vi "voltage phase conv SM.vi"() -> ()   [LabVIEW 2019]
uses:
  <vilib>/Utility/file.llb/Write Delimited Spreadsheet (DBL).vi
panel:
  in  "Stop Button":bool
  out "Current pixel":dbl=591.0
  in  "Max pixel":i32=590
  in  "Mask B Calibration Path":path=path "G:/My Drive/ansom/Data/THz 1/pulse shaping/SLM voltage calibration 20 July 2021/Mask B voltage transmission.txt"
  in  "Mask A Calibration Path":path=path "G:/My Drive/ansom/Data/THz 1/pulse shaping/SLM voltage calibration 20 July 2021/Mask A voltage transmission.txt"
  in  "Mask B Data folder":path=path "G:/My Drive/ansom/Data/THz 1/pulse shaping/SLM voltage calibration 20 July 2021/Mask_B_phase_voltage"
  in  "Mask A Data folder":path=path "G:/My Drive/ansom/Data/THz 1/pulse shaping/SLM voltage calibration 20 July 2021/Mask_A_phase_voltage"
  in  "Starting pixel":dbl=518.0 format="%#_13g"
  in  "START":bool
  # "Inputs"
  # "Insert file paths to SLM calibration output .txt files"
  # "Insert folder paths to tell the program where to save voltage/phase .txt files"
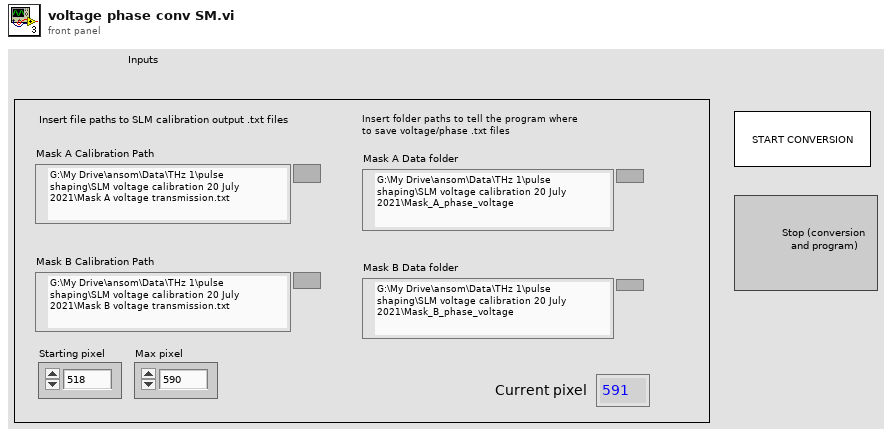
[diagram p1: front panel]
types:
  T1 = enum32{"Invalid", "Standard", "Closed", "Hidden", "Minimized", "Maximized"}
  T2 = enum32{"invalid app kind", "Development System", "Run Time System", "Student Edition", "Embedded LabVIEW", "Evaluation", "Custom"}
  T3 = cluster{"Core":cluster{"Current VI Reference":refnum<vi>, "Close Panel on Exit?":bool}, "Your Boolean data":bool, "Your string data":string}
  T4 = cluster{"Current VI Reference":refnum<vi>, "Close Panel on Exit?":bool}
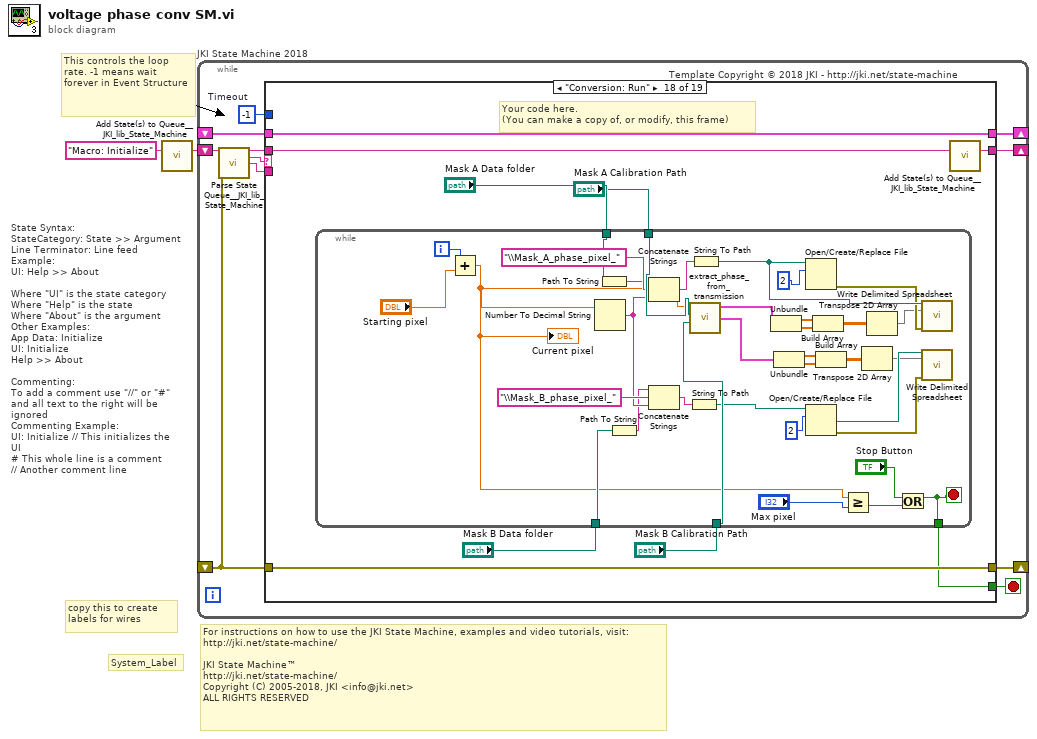
[diagram p0: block diagram]
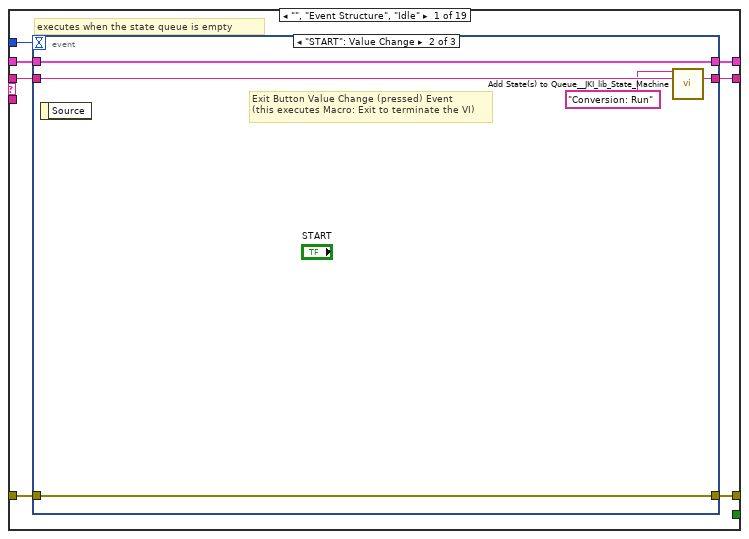
[diagram p2: hidden frame]
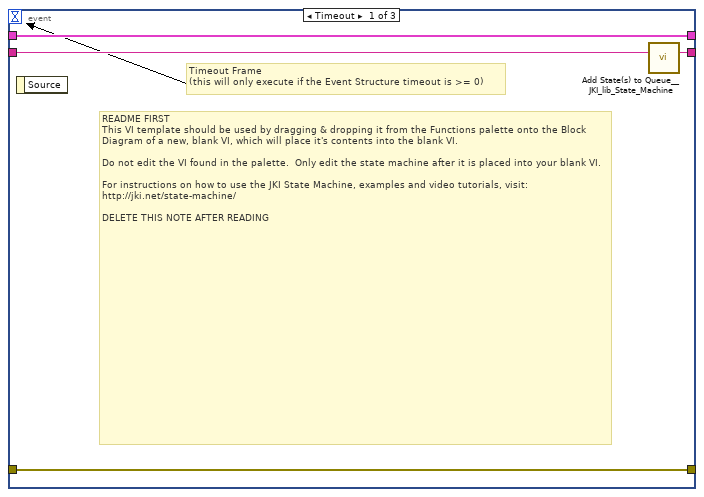
[diagram p3: hidden frame]
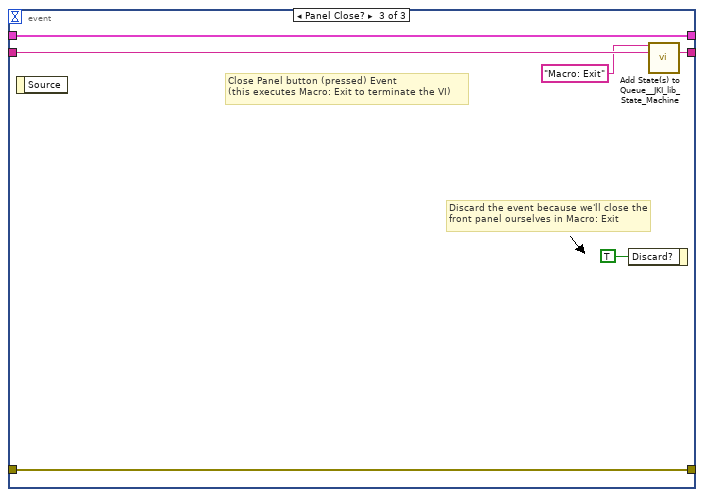
[diagram p4: hidden frame]
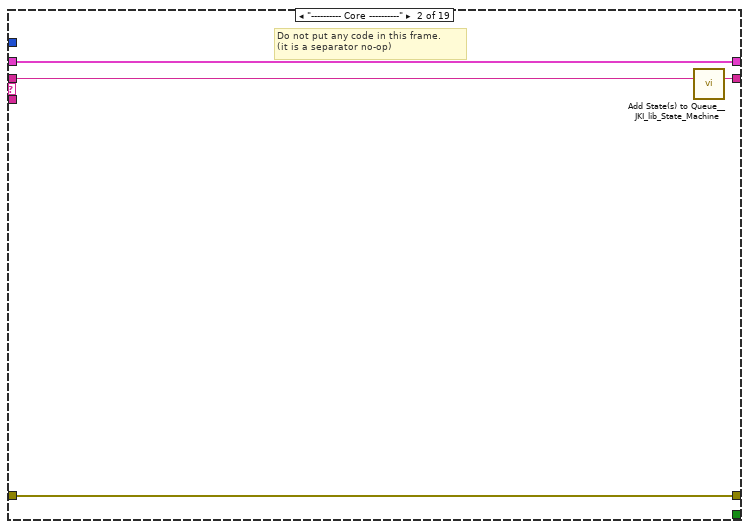
[diagram p5: hidden frame]
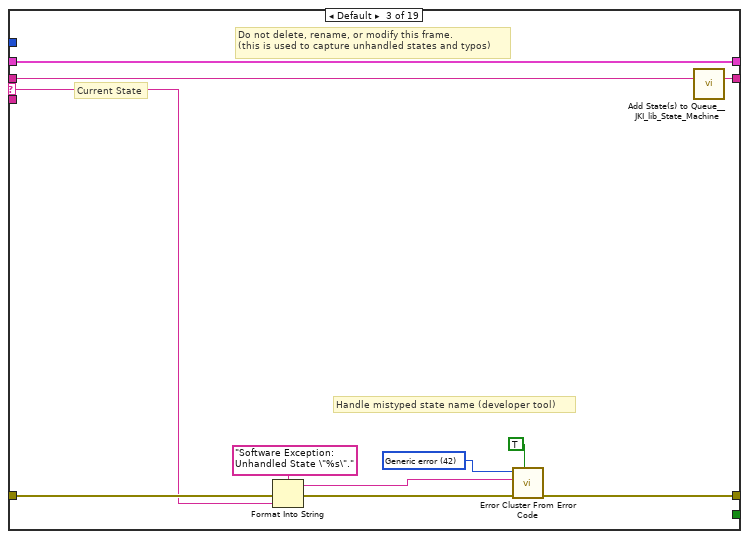
[diagram p6: hidden frame]
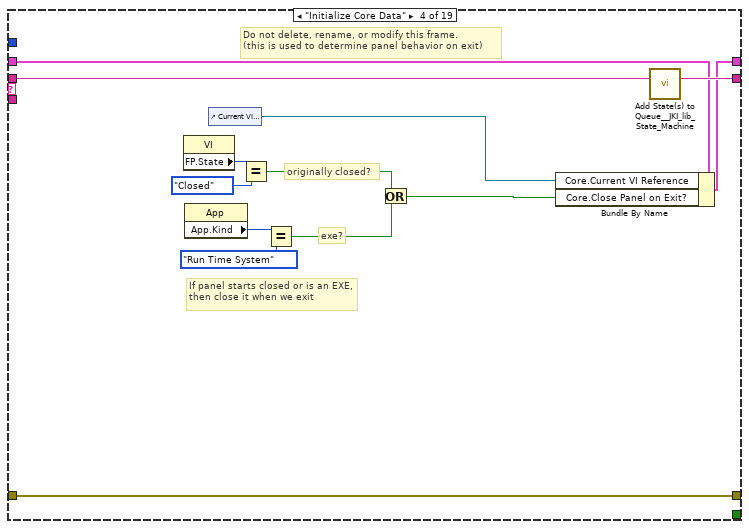
[diagram p7: hidden frame]
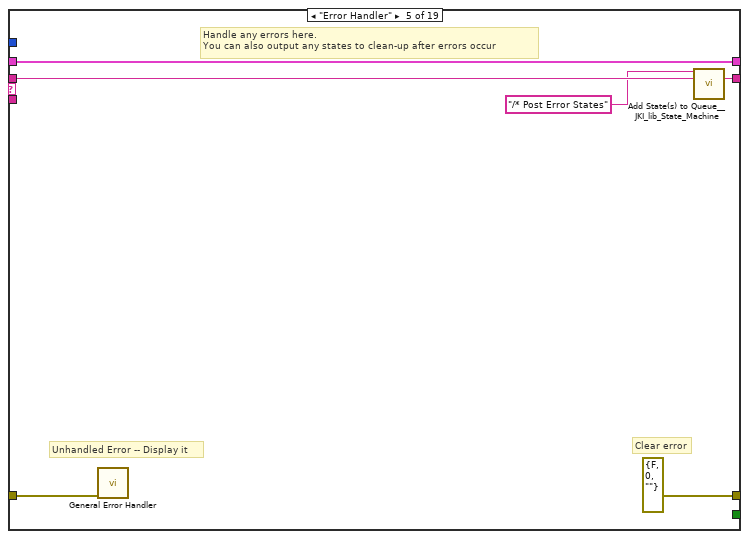
[diagram p8: hidden frame]
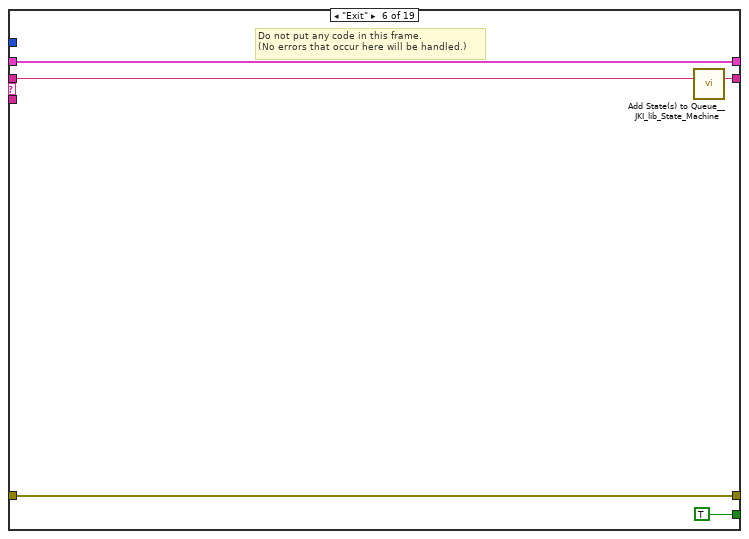
[diagram p9: hidden frame]
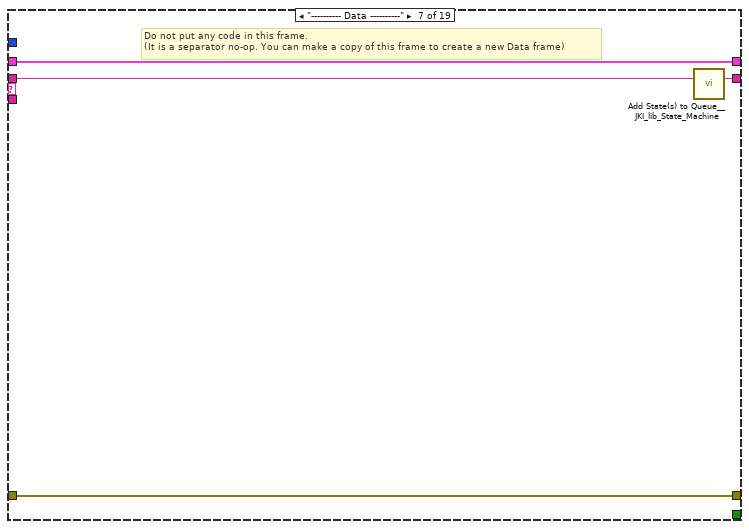
[diagram p10: hidden frame]
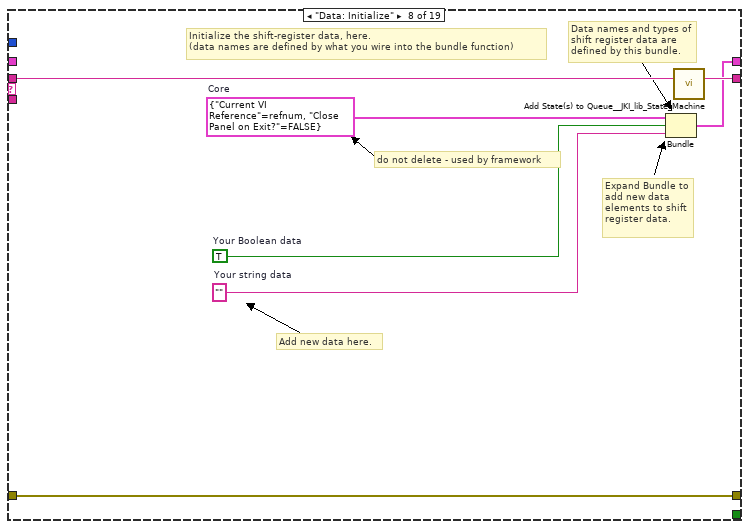
[diagram p11: hidden frame]
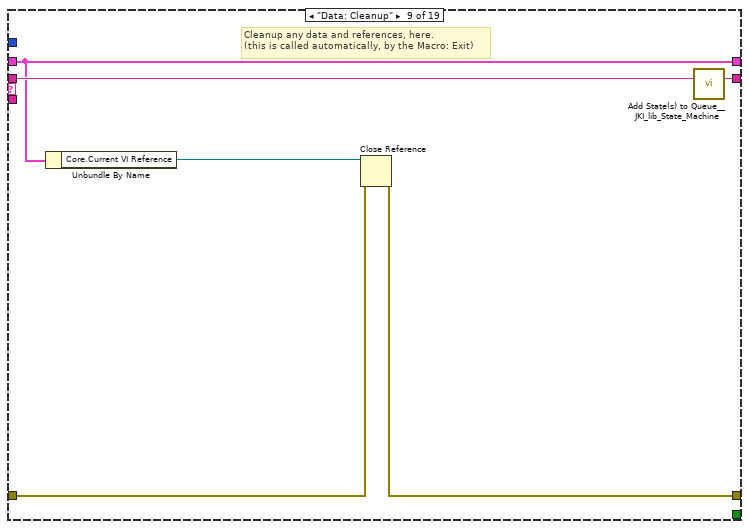
[diagram p12: hidden frame]
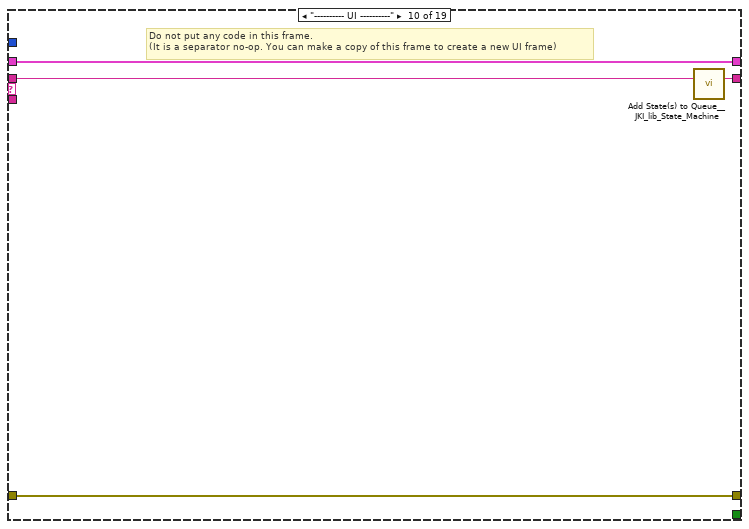
[diagram p13: hidden frame]
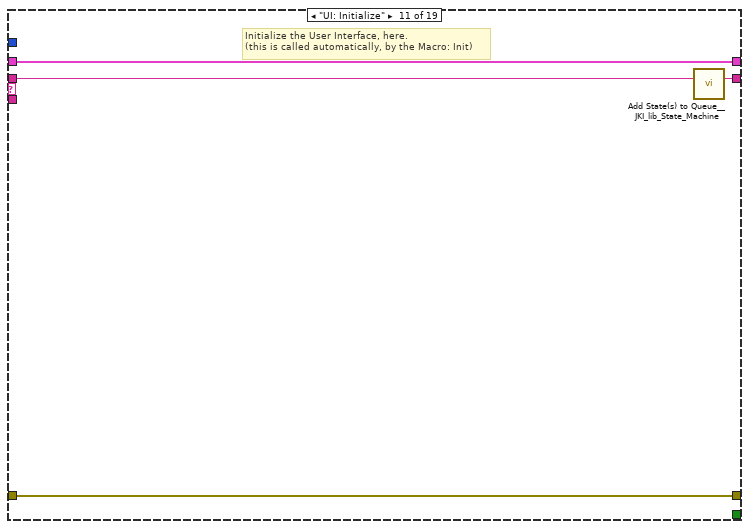
[diagram p14: hidden frame]
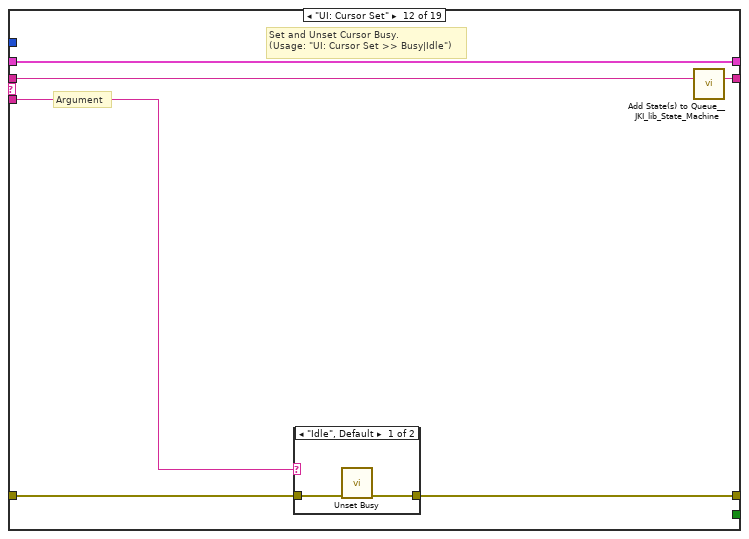
[diagram p15: hidden frame]
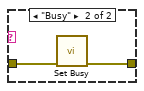
[diagram p16: hidden frame]
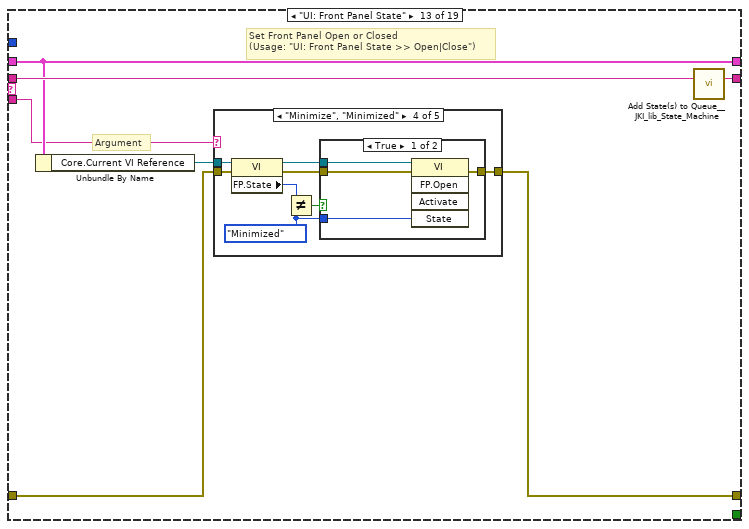
[diagram p17: hidden frame]
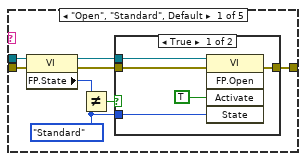
[diagram p18: hidden frame]
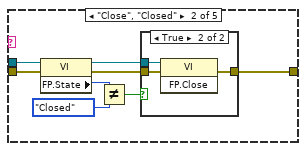
[diagram p20: hidden frame]
diagram:
  # "For instructions on how to use the JKI State Machine, examples and video tutorials, visit:\nhttp://jki.net/state-machine/\n\nJKI State Machine™\nhttp://jki.net/state-machine/\nCopyright (C) 2005-2018, JKI <info@jki.net>\nALL RIGHTS RESERVED"
  # "State Syntax:\nStateCategory: State >> Argument\nLine Terminator: Line feed\nExample:\nUI: Help >> About\n\nWhere \"UI\" is the state category\nWhere \"Help\" is the state\nWhere \"About\" is the argument\nOther Examples:\nApp Data: Initialize\nUI: Initialize\nHelp >> About\n\nCommenting:\nTo add a comment use \"//\" or \"#\" and all text to the right will be ignored\nCommenting Example:\nUI: Initialize // This initializes the UI\n# This whole line is a comment\n// Another comment line"
  # "copy this to create labels for wires"
  # "This controls the loop rate. -1 means wait forever in Event Structure"
  # "System_Label"
  n1 = call <vilib>:"Add State(s) to Queue__JKI_lib_State_Machine.vi"("State(s) in (\"\")"="Macro: Initialize") -> ("States Out"=w2:string)  [unwired: 14 in]
  n2 = while "JKI State Machine 2018" {
    shift-right: [w6] -> _
    shift-left: _ -> [w5]
    shift-right: [w9] -> _
    shift-left: _ -> [w3]
    shift-right: [w8] -> _
    shift-left: w2 -> [w10]
    stop <- w7 stop-if-true
    w4 = -1  # Timeout
    # "Template Copyright © 2018 JKI - http://jki.net/state-machine"
    n3 = call <vilib>:"Parse State Queue__JKI_lib_State_Machine.vi"("State Queue"=w10, "Error In (no error)"=w3) -> ("Remaining States"=w12:string, "Current State"=w13:string, "Arguments"=w11:string)  [unwired: 11 in]
    n4 = case shown="\"Conversion: Run\"" w13 {
      selector: w13 -> [_ _ w40 _ _ _ _ _ _ _ _ _ _ _ _ _ _ _ _]
      tunnel: w12 -> [w20 w39 w44 w63 w69 w74 w78 w85 w91 w95 w99 w105 w116 w185 w190 w200 w204 w213 w251]
      tunnel: w11 -> [_ _ _ _ _ _ _ _ _ _ _ w100 w110 _ _ _ _ _ _]
      tunnel: w5 -> [w18 w36 w42 w56 w66 w72 w75 _ w86 w92 w97 w103 w112 w182 w187 w197 w201 w210 w248]
      tunnel: [w17 w37 w46 w60 errorcluster {"status"=FALSE, "code"=0, "source"=""} ("error out") w71 w76 w82 w87 w93 w96 w101 w113 w183 w188 w198 w202 w211 w249] -> w9
      tunnel: w3 -> [w16 w37 w45 w60 w65 w71 w76 w82 w88 w93 w96 w102 w114 w183 w188 w198 w202 w211 w249]
      tunnel: [w19 w38 w43 w62 w68 w73 w77 w84 w90 w94 w98 w104 w115 w184 w189 w199 w203 w212 w250] -> w8
      tunnel: [_ _ _ _ _ TRUE _ _ _ _ _ _ _ _ _ _ _ w205 _] -> w7
      tunnel: [w15 w36 w42 w61 w66 w72 w75 w83 w86 w92 w97 w103 w112 w182 w187 w197 w201 w210 w248] -> w6
      tunnel: w4 -> [w14 _ _ _ _ _ _ _ _ _ _ _ _ _ _ _ _ _ _]
      frame "", "Event Structure", "Idle" {
        # "executes when the state queue is empty"
        n5 = event shown="[1] \"START\": Value Change" {
          selector: _ -> [_ _ _]
          dyn-events: _ -> [_ _ _]
          timeout: w14 -> [_ _ _]
          tunnel: w20 -> [w24 w29 w35]
          tunnel: [w23 w28 w34] -> w19
          tunnel: w18 -> [w21 w26 w32]
          tunnel: [w22 w27 w33] -> w17
          tunnel: w16 -> [w22 w27 w33]
          tunnel: [w21 w26 w32] -> w15
          event Timeout {
            # "README FIRST\nThis VI template should be used by dragging & dropping it from the Functions palette onto the Block Diagram of a new, blank VI, which will place it's contents into the blank VI.\n\nDo not edit the VI found in the palette.  Only edit the state machine after it is placed into your blank VI.\n\nFor instructions on how to use the JKI State Machine, examples and video tutorials, visit:\nhttp://jki.net/state-machine/\n\nDELETE THIS NOTE AFTER READING"
            # "Timeout Frame\n(this will only execute if the Event Structure timeout is >= 0)"
            n6 = event-data() -> ()  [unwired: 1 in, 1 out]
            n7 = call <vilib>:"Add State(s) to Queue__JKI_lib_State_Machine.vi"("State(s) in (\"\")"=w24) -> ("States Out"=w23:string)  [unwired: 14 in]
          }
          event "START": Value Change {
            # "Exit Button Value Change (pressed) Event\n(this executes Macro: Exit to terminate the VI)"
            n8 = event-data() -> ()  [unwired: 1 in, 1 out]
            n9 = call <vilib>:"Add State(s) to Queue__JKI_lib_State_Machine.vi"("State(s) in Front (\"\")"="Conversion: Run", "State(s) in (\"\")"=w29) -> ("States Out"=w28:string)  [unwired: 13 in]
          }
          event Panel Close? {
            # "Discard the event because we'll close the front panel ourselves in Macro: Exit"
            # "Close Panel button (pressed) Event\n(this executes Macro: Exit to terminate the VI)"
            n10 = event-data() -> ()  [unwired: 1 in, 1 out]
            n11 = event-data("Discard?"=TRUE) -> ()  [unwired: 1 in, 1 out]
            n12 = call <vilib>:"Add State(s) to Queue__JKI_lib_State_Machine.vi"("State(s) in Front (\"\")"="Macro: Exit", "State(s) in (\"\")"=w35) -> ("States Out"=w34:string)  [unwired: 13 in]
          }
        }
      }
      frame "---------- Core ----------" {
        # "Do not put any code in this frame.\n(it is a separator no-op)"
        n13 = call <vilib>:"Add State(s) to Queue__JKI_lib_State_Machine.vi"("State(s) in (\"\")"=w39) -> ("States Out"=w38:string)  [unwired: 14 in]
      }
      frame Default {
        w49 = 42 items=["No error", "Argument error", "Memory is full", "Out of zone", "End of file", "File already open", "Generic file I/O error", "File not found", "File permission error", "Disk is full", "Duplicate path", "Too many files open", "System feature not enabled", "Resource file not found", "Cannot add resource", "Resource not found", "Image not found", "Image memory error", "Pen does not exist", "Config type invalid", "Config token not found", "Config parse error", "Config memory error", "Bad external code format", "Bad external code offset", "External code not present", "Null window", "Destroy window error", "Null menu", "Print aborted", "Bad print record", "Print driver error", "Windows error during printing", "Memory error during printing", "Print dialog error", "Generic print error", "Invalid device refnum", "Device not found", "Device parameter error", "Device unit error", "Cannot open device", "Device call aborted", "Generic error", "Cancelled by user", "Object ID too low", "Object ID too high", "Object not in heap", "Unknown heap", "Unknown object (invalid DefProc)", "Unknown object (DefProc not in table)", "Message out of range", "Invalid (null) method", "Unknown message", "Manager call not supported", "Bad address", "Network operation in progress", "Network operation timed out", "Connection is busy", "Network attribute not supported", "Network error", "Address in use", "System out of memory", "Connection aborted", "Connection refused", "Not connected", "Already connected", "Connection closed", "Initialization error (interapplication manager)", "Bad occurrence", "Wait on unbound occurrence handler", "Occurrence queue overflow", "Datalog type conflict", "Unused", "Unrecognized type (interapplication manager)", "Memory corrupt", "Failed to make temporary DLL", "Old CIN version", "Drag socket not found", "Failed to load drop-object", "Failed to register OLE object", "Failed to release OLE object", "Format specifier type mismatch", "Unknown format specifier", "Too few format specifiers", "Too many format specifiers", "Scan failed", "Newer CIN version", "Error converting to variant", "Runtime menu error", "Password tampered", "Variant attribute not found", "Incompatible variant data type", "Event data is not available", "Event Store is not present", "Occurrence is not found", "Event Queue is not created", "Event info is not available", "Refnum passed is NULL", "Error retrieving Class GUID", "Error retrieving CoClass GUID", "Error retrieving TypeLib GUID.", "Bad built application magic bytes.", "Specific driver is different from the specific driver associated with the Logical Name.", "There is no session opened to the class driver.", "Max Error", "MAX - Error with config objects", "MAX - Error loading configuration", "MAX - Group not supported"]
        # "Current State"
        # "Do not delete, rename, or modify this frame.\n(this is used to capture unhandled states and typos)"
        # "Handle mistyped state name (developer tool)"
        n14 = Format Into String(format string="Software Exception: Unhandled State \"%s\"." ("message"), error in=w45, w40) -> (resulting string=w48:string, error out=w47:errorcluster)  [unwired: 1 in]
        n15 = call <vilib>:"Error Cluster From Error Code.vi"("show call chain? (False)"=TRUE, "error in (no error)"=w47, "error message (\"\")"=w48, "error code (0)"=w49) -> ("error out"=w46:errorcluster)  [unwired: 5 in]
        n16 = call <vilib>:"Add State(s) to Queue__JKI_lib_State_Machine.vi"("State(s) in (\"\")"=w44) -> ("States Out"=w43:string)  [unwired: 14 in]
      }
      frame "Initialize Core Data" {
        # "Do not delete, rename, or modify this frame.\n(this is used to determine panel behavior on exit)"
        # "originally closed?"
        # "exe?"
        # "If panel starts closed or is an EXE, then close it when we exit"
        n17 = property class="VI"() -> ("FP.State"=w53:T1)  [unwired: 2 in, 2 out]
        n18 = property class="App"() -> ("App.Kind"=w59:T2)  [unwired: 2 in, 2 out]
        n19 = control-ref of="Current VI Reference"() -> (w54:refnum<vi>)
        n20 = Equal?(x=w53, y=T1."Closed" ("Front Panel Window:State")) -> (x = y?=w51:bool)
        n21 = Equal?(x=w59, y=T2."Run Time System" ("Application:Kind")) -> (x = y?=w57:bool)
        n22 = Or(x=w51, y=w57) -> (x .or. y?=w55:bool)
        n23 = Bundle By Name(cluster=w56, "Core.Current VI Reference"=w54, "Core.Close Panel on Exit?"=w55) -> (w61:T3)
        n24 = call <vilib>:"Add State(s) to Queue__JKI_lib_State_Machine.vi"("State(s) in (\"\")"=w63) -> ("States Out"=w62:string)  [unwired: 14 in]
      }
      frame "Error Handler" {
        # "Unhandled Error -- Display it"
        # "Handle any errors here.\nYou can also output any states to clean-up after errors occur"
        # "Clear error"
        n25 = call <vilib>:"General Error Handler.vi"("error in (no error)"=w65) -> ()  [unwired: 10 in, 5 out]
        n26 = call <vilib>:"Add State(s) to Queue__JKI_lib_State_Machine.vi"("State(s) in Front (\"\")"="/* Post Error States", "State(s) in (\"\")"=w69) -> ("States Out"=w68:string)  [unwired: 13 in]
      }
      frame "Exit" {
        # "Do not put any code in this frame.\n(No errors that occur here will be handled.)"
        n27 = call <vilib>:"Add State(s) to Queue__JKI_lib_State_Machine.vi"("State(s) in (\"\")"=w74) -> ("States Out"=w73:string)  [unwired: 14 in]
      }
      frame "---------- Data ----------" {
        # "Do not put any code in this frame.\n(It is a separator no-op. You can make a copy of this frame to create a new Data frame)"
        n28 = call <vilib>:"Add State(s) to Queue__JKI_lib_State_Machine.vi"("State(s) in (\"\")"=w78) -> ("States Out"=w77:string)  [unwired: 14 in]
      }
      frame "Data: Initialize" {
        w79 = T4 {"Current VI Reference"=refnum, "Close Panel on Exit?"=FALSE}  # Core
        w81 = TRUE  # Your Boolean data
        w80 = ""  # Your string data
        # "do not delete - used by framework"
        # "Expand Bundle to add new data elements to shift register data."
        # "Add new data here."
        # "Data names and types of shift register data are defined by this bundle."
        # "Initialize the shift-register data, here.\n(data names are defined by what you wire into the bundle function)"
        n29 = Bundle("Core"=w79, "Your Boolean data"=w81, "Your string data"=w80) -> (w83:T3)  [unwired: 1 in]
        n30 = call <vilib>:"Add State(s) to Queue__JKI_lib_State_Machine.vi"("State(s) in (\"\")"=w85) -> ("States Out"=w84:string)  [unwired: 14 in]
      }
      frame "Data: Cleanup" {
        # "Cleanup any data and references, here.\n(this is called automatically, by the Macro: Exit)"
        n31 = Unbundle By Name(w86) -> ("Core.Current VI Reference"=w89:refnum<vi>)
        n32 = Close Reference(reference=w89, error in (no error)=w88) -> (error out=w87:errorcluster)
        n33 = call <vilib>:"Add State(s) to Queue__JKI_lib_State_Machine.vi"("State(s) in (\"\")"=w91) -> ("States Out"=w90:string)  [unwired: 14 in]
      }
      frame "---------- UI ----------" {
        # "Do not put any code in this frame.\n(It is a separator no-op. You can make a copy of this frame to create a new UI frame)"
        n34 = call <vilib>:"Add State(s) to Queue__JKI_lib_State_Machine.vi"("State(s) in (\"\")"=w95) -> ("States Out"=w94:string)  [unwired: 14 in]
      }
      frame "UI: Initialize" {
        # "Initialize the User Interface, here.\n(this is called automatically, by the Macro: Init)"
        n35 = call <vilib>:"Add State(s) to Queue__JKI_lib_State_Machine.vi"("State(s) in (\"\")"=w99) -> ("States Out"=w98:string)  [unwired: 14 in]
      }
      frame "UI: Cursor Set" {
        # "Argument"
        # "Set and Unset Cursor Busy.\n(Usage: \"UI: Cursor Set >> Busy|Idle\")"
        n36 = case shown="\"Idle\", Default" w100 {
          tunnel: w102 -> [w107 w109]
          tunnel: [w106 w108] -> w101
          frame "Idle", Default {
            n37 = call <vilib>:"Unset Busy.vi"("error in (no error)"=w107) -> ("error out"=w106:errorcluster)  [unwired: 10 in]
          }
          frame "Busy" {
            n38 = call <vilib>:"Set Busy.vi"("error in (no error)"=w109) -> ("error out"=w108:errorcluster)  [unwired: 9 in, 1 out]
          }
        }
        n39 = call <vilib>:"Add State(s) to Queue__JKI_lib_State_Machine.vi"("State(s) in (\"\")"=w105) -> ("States Out"=w104:string)  [unwired: 14 in]
      }
      frame "UI: Front Panel State" {
        # "Argument"
        # "Set Front Panel Open or Closed\n(Usage: \"UI: Front Panel State >> Open|Close\")"
        n40 = Unbundle By Name(w112) -> ("Core.Current VI Reference"=w111:refnum<vi>)
        n41 = case shown="\"Minimize\", \"Minimized\"" w110 {
          tunnel: w114 -> [w122 w137 w148 w161 w174]
          tunnel: [w124 w138 w150 w163 w176] -> w113
          tunnel: w111 -> [w123 w135 w149 w162 w175]
          frame "Open", "Standard", Default {
            w117 = T1."Standard" ("State")
            n42 = property class="VI"(reference=w123, error in=w122) -> (reference out=w120:refnum<vi>, error out=w121:errorcluster, "FP.State"=w119:T1)
            n43 = Not Equal?(x=w119, y=w117) -> (x != y?=w118:bool)
            n44 = case shown="True" w118 {
              tunnel: [w128 w130] -> w124
              tunnel: w121 -> [w127 w130]
              tunnel: w120 -> [w126 _]
              tunnel: w117 -> [w125 _]
              frame True {
                n45 = invoke class="VI" method="FP.Open"(reference=w126, error in=w127, "Activate"=TRUE, "State"=w125) -> (error out=w128:errorcluster)  [unwired: 1 in, 4 out]
              }
              frame False {
              }
            }
          }
          frame "Close", "Closed" {
            n46 = property class="VI"(reference=w135, error in=w137) -> (reference out=w134:refnum<vi>, error out=w136:errorcluster, "FP.State"=w132:T1)
            n47 = Not Equal?(x=w132, y=T1."Closed" ("Front Panel Window:State")) -> (x != y?=w131:bool)
            n48 = case shown="True" w131 {
              tunnel: [w139 w142] -> w138
              tunnel: w136 -> [w139 w141]
              tunnel: w134 -> [_ w140]
              frame False {
              }
              frame True {
                n49 = invoke class="VI" method="FP.Close"(reference=w140, error in=w141) -> (error out=w142:errorcluster)  [unwired: 1 in, 2 out]
              }
            }
          }
          frame "Hidden", "Hide" {
            w143 = T1."Hidden" ("State")
            n50 = property class="VI"(reference=w149, error in=w148) -> (reference out=w146:refnum<vi>, error out=w147:errorcluster, "FP.State"=w145:T1)
            n51 = Not Equal?(x=w145, y=w143) -> (x != y?=w144:bool)
            n52 = case shown="True" w144 {
              tunnel: [w154 w155] -> w150
              tunnel: w147 -> [w153 w155]
              tunnel: w146 -> [w152 _]
              tunnel: w143 -> [w151 _]
              frame True {
                n53 = invoke class="VI" method="FP.Open"(reference=w152, error in=w153, "State"=w151) -> (error out=w154:errorcluster)  [unwired: 2 in, 4 out]
              }
              frame False {
              }
            }
          }
          frame "Minimize", "Minimized" {
            w156 = T1."Minimized" ("State")
            n54 = property class="VI"(reference=w162, error in=w161) -> (reference out=w159:refnum<vi>, error out=w160:errorcluster, "FP.State"=w158:T1)
            n55 = Not Equal?(x=w158, y=w156) -> (x != y?=w157:bool)
            n56 = case shown="True" w157 {
              tunnel: [w167 w168] -> w163
              tunnel: w160 -> [w166 w168]
              tunnel: w159 -> [w165 _]
              tunnel: w156 -> [w164 _]
              frame True {
                n57 = invoke class="VI" method="FP.Open"(reference=w165, error in=w166, "State"=w164) -> (error out=w167:errorcluster)  [unwired: 2 in, 4 out]
              }
              frame False {
              }
            }
          }
          frame "Maximize", "Maximized" {
            w169 = T1."Maximized" ("State")
            n58 = property class="VI"(reference=w175, error in=w174) -> (reference out=w172:refnum<vi>, error out=w173:errorcluster, "FP.State"=w171:T1)
            n59 = Not Equal?(x=w171, y=w169) -> (x != y?=w170:bool)
            n60 = case shown="True" w170 {
              tunnel: [w180 w181] -> w176
              tunnel: w173 -> [w179 w181]
              tunnel: w172 -> [w178 _]
              tunnel: w169 -> [w177 _]
              frame True {
                n61 = invoke class="VI" method="FP.Open"(reference=w178, error in=w179, "State"=w177) -> (error out=w180:errorcluster)  [unwired: 2 in, 4 out]
              }
              frame False {
              }
            }
          }
        }
        n62 = call <vilib>:"Add State(s) to Queue__JKI_lib_State_Machine.vi"("State(s) in (\"\")"=w116) -> ("States Out"=w115:string)  [unwired: 14 in]
      }
      frame "---------- Macro ----------" {
        # "Do not put any code in this frame.\n(It is a separator no-op. You can make a copy of this frame to create a new Macro frame)"
        n63 = call <vilib>:"Add State(s) to Queue__JKI_lib_State_Machine.vi"("State(s) in (\"\")"=w185) -> ("States Out"=w184:string)  [unwired: 14 in]
      }
      frame "Macro: Initialize" {
        w186 = "Data: Initialize\nInitialize Core Data\nUI: Initialize\nUI: Front Panel State >> Open"  # Data: Initialize Initialize Core Data UI: Initialize UI: Front Panel State >> Open
        # "Initialization Macro\n(This is called once, when the VI starts)"
        n64 = call <vilib>:"Add State(s) to Queue__JKI_lib_State_Machine.vi"("State(s) in Front (\"\")"=w186, "State(s) in (\"\")"=w190) -> ("States Out"=w189:string)  [unwired: 13 in]
      }
      frame "Macro: Exit" {
        # "Exit Macro\n(This is called once, when the VI exits)"
        n65 = Unbundle By Name(w197) -> ("Core.Close Panel on Exit?"=w196:bool)
        n66 = Select(t="UI: Front Panel State >> Close", s=w196, f="") -> (s? t:f=w193:string)
        n67 = call <vilib>:"Add State(s) to Queue__JKI_lib_State_Machine.vi"("State(s) in (\"\")"=w193, "State(s) at Back (\"\")"="Data: Cleanup\nExit") -> ("States Out"=w191:string)  [unwired: 13 in]
        n68 = call <vilib>:"Add State(s) to Queue__JKI_lib_State_Machine.vi"("State(s) in Front (\"\")"=w191, "State(s) in (\"\")"=w200) -> ("States Out"=w199:string)  [unwired: 13 in]
      }
      frame "---------- New Category ----------" {
        # "Template Separator\n(You can make a copy of, or modify, this frame)"
        n69 = call <vilib>:"Add State(s) to Queue__JKI_lib_State_Machine.vi"("State(s) in (\"\")"=w204) -> ("States Out"=w203:string)  [unwired: 14 in]
      }
      frame "Conversion: Run" {
        # "Your code here.\n(You can make a copy of, or modify, this frame)"
        n70 = while {
          tunnel: "Mask A Data folder" -> [w246]
          tunnel: "Mask B Data folder" -> [w245]
          tunnel: "Mask A Calibration Path" -> [w244]
          tunnel: "Mask B Calibration Path" -> [w243]
          tunnel: [w226] -> w205
          i -> [w247]
          stop <- w226 stop-if-true
          n71 = Add(x=w247, y="Starting pixel") -> (x+y=w227:dbl)
          "Current pixel" <- w227
          n72 = Number To Decimal String(number=w227) -> (decimal integer string=w238:string)  [unwired: 1 in]
          n73 = Path To String(path=w246) -> (string=w237:string)
          n74 = Path To String(path=w245) -> (string=w232:string)
          n75 = Concatenate Strings(w237, "\\Mask_A_phase_pixel_", w238) -> (w242:string)
          n76 = Concatenate Strings(w232, "\\Mask_B_phase_pixel_", w238) -> (w235:string)
          n77 = String To Path(string=w235) -> (path=w233:path)
          n78 = call "extract_phase_from_transmission.vi"("Mask B Calibration Path"=w243, "Mask A Calibration Path"=w244, "Pixel number"=w227) -> ("Mask B Phase"=w236:cluster{"Ramp Pattern":dbl[], "phase out":dbl[]}, "Mask A Phase"=w240:cluster{"Ramp Pattern":dbl[], "phase out":dbl[]})  [unwired: 7 in]
          n79 = String To Path(string=w242) -> (path=w234:path)
          n80 = Unbundle(w240) -> ("Ramp Pattern"=w224:dbl[], "phase out"=w223:dbl[])
          n81 = Unbundle(w236) -> ("Ramp Pattern"=w222:dbl[], "phase out"=w221:dbl[])
          n82 = Open/Create/Replace File(file path (use dialog)=w234, operation (0:open)=2) -> (error out=w220:errorcluster)  [unwired: 4 in, 2 out]
          n83 = Open/Create/Replace File(file path (use dialog)=w233, operation (0:open)=2) -> (error out=w219:errorcluster)  [unwired: 4 in, 2 out]
          n84 = Build Array(w224, w223) -> (w216:dbl[][])
          n85 = Build Array(w222, w221) -> (w217:dbl[][])
          n86 = Greater Or Equal?(x=w227, y="Max pixel") -> (x >= y?=w229:bool)
          n87 = Transpose 2D Array(2D array=w217) -> (transposed array=w214:dbl[][])
          n88 = Transpose 2D Array(2D array=w216) -> (transposed array=w215:dbl[][])
          n89 = Or(x="Stop Button", y=w229) -> (x .or. y?=w226:bool)
          n90 = call-poly <vilib>:"Write Delimited Spreadsheet.vi"("file path (dialog if empty)"=w234, "2D data"=w215, "error in (no error)"=w220) -> ()  [unwired: 11 in, 2 out]
          n91 = call-poly <vilib>:"Write Delimited Spreadsheet.vi"("file path (dialog if empty)"=w233, "2D data"=w214, "error in (no error)"=w219) -> ()  [unwired: 11 in, 2 out]
        }
        n92 = call <vilib>:"Add State(s) to Queue__JKI_lib_State_Machine.vi"("State(s) in (\"\")"=w213) -> ("States Out"=w212:string)  [unwired: 14 in]
      }
      frame "New Category: 2" {
        # "Your code here.\n(You can make a copy of, or modify, this frame)"
        n93 = call <vilib>:"Add State(s) to Queue__JKI_lib_State_Machine.vi"("State(s) in (\"\")"=w251) -> ("States Out"=w250:string)  [unwired: 14 in]
      }
    }
  }
